vi "SetTrigger.vi"(1 "TriggerSettings":T1, 2 "deviceNumber":i32) -> (0 "success":i32)   [LabVIEW 2009]
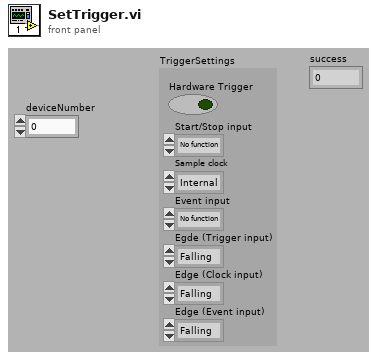
[diagram p1: front panel]
types:
  T1 = cluster{"Hardware Trigger":bool, "Start/Stop input":enum32{"No function", "Start trigger", "Start/Stop trigger", "Start/Stop processed"}, "Sample clock":enum32{"Internal", "External"}, "Event input":enum32{"No function", "Single value"}, "Egde (Trigger input)":enum32{"Falling", "Rising"}, "Edge (Clock input)":enum32{"Falling", "Rising"}, "Edge (Event input)":enum32{"Falling", "Rising"}}
  T2 = enum32{"No function", "Start trigger", "Start/Stop trigger", "Start/Stop processed"}
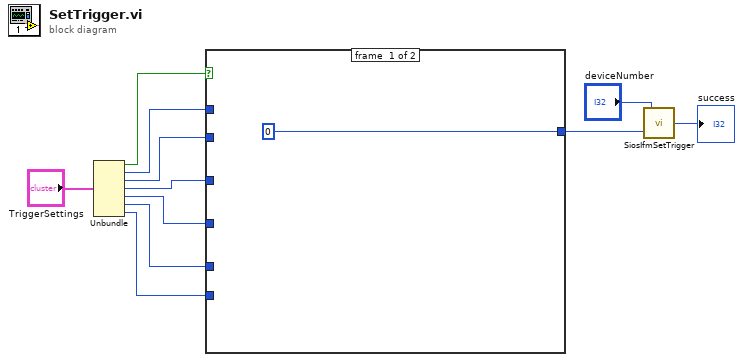
[diagram p0: block diagram]
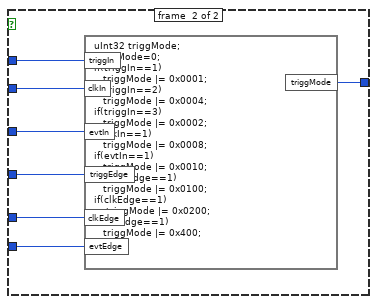
[diagram p2: hidden frame]
diagram:
  n1 = Unbundle("TriggerSettings") -> ("Hardware Trigger"=w5:bool, "Start/Stop input"=w6:T2, "Sample clock"=w7:enum32{"Internal", "External"}, "Event input"=w8:enum32{"No function", "Single value"}, "Egde (Trigger input)"=w9:enum32{"Falling", "Rising"}, "Edge (Clock input)"=w11:enum32{"Falling", "Rising"}, "Edge (Event input)"=w10:enum32{"Falling", "Rising"})
  n2 = case shown="True" w5 {
    tunnel: [u32 0 w19] -> w2
    tunnel: w6 -> [_ w18]
    tunnel: w7 -> [_ w17]
    tunnel: w8 -> [_ w16]
    tunnel: w9 -> [_ w15]
    tunnel: w10 -> [_ w14]
    tunnel: w11 -> [_ w13]
    frame #0 {
    }
    frame #1 {
      n3 = formula code="uInt32 triggMode;\ntriggMode=0;\nif(triggIn==1)\n   triggMode |= 0x0001;\nif(triggIn==2)\n   triggMode |= 0x0004;\nif(triggIn==3)\n   triggMode |= 0x0002;\nif(clkIn==1)\n   triggMode |= 0x0008;\nif(evtIn==1)\n   triggMode |= 0x0010;\nif(triggEdge==1)\n   triggMode |= 0x0100;\nif(clkEdge==1)\n    triggMode |= 0x0200;\nif(evtEdge==1)\n   triggMode |= 0x400;"("triggIn"=w18, "clkIn"=w17, "evtIn"=w16, "triggEdge"=w15, "clkEdge"=w13, "evtEdge"=w14) -> ("triggMode"=w19:u32)
    }
  }
  n4 = call "SiosIfmSetTrigger.vi"("triggerMode"=w2, "devNumber"="deviceNumber") -> ("success"=→"success":i32)
